vi "create_method.vi"(0 "template_path":path=path "C:/Users/hugoc/TDF Dropbox/2_Technologies de France/1 - Services et Etudes/_Missions/HC/6 - PLAIYLAB/code/Model/_Template/common/specific_data/fit.vit", 5 "ModuleModelFunction":string[](array[string])=["tree", "DecisionTreeClassifier", "fit"], 7 "Control Path":path=path "C:/Users/hugoc/TDF Dropbox/2_Technologies de France/1 - Services et Etudes/_Missions/HC/6 - PLAIYLAB/code/Model/Supervised/Tree/Tree.lvclass", 9 "Path to Saved File":path, 11 "error in (no error)":errorcluster, 12 "Parameters?":bool) -> (15 "error out":errorcluster)   [LabVIEW 2020]
doc: "Create a method based on a template with the correct documentation."
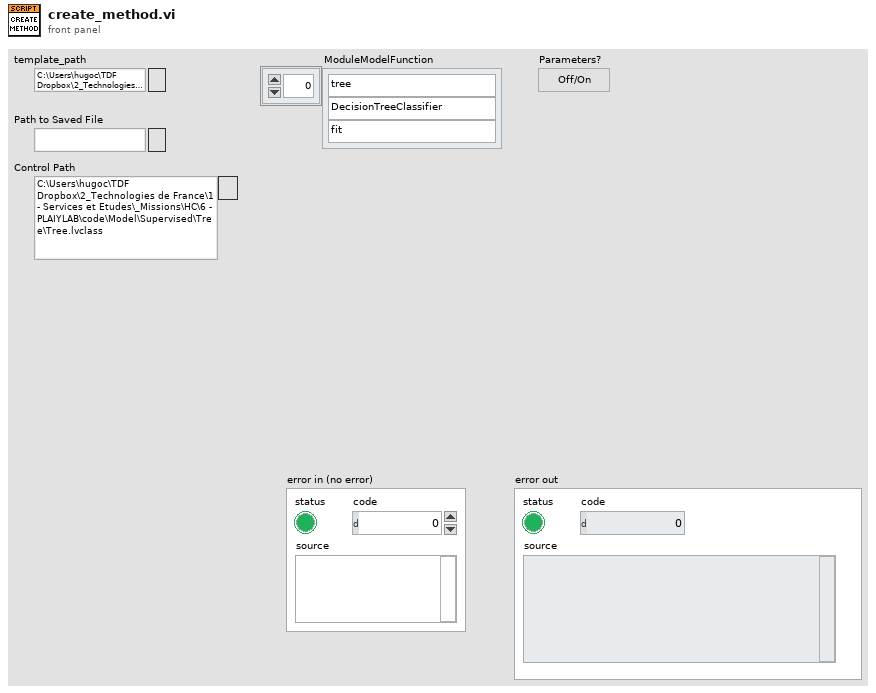
[diagram p1: front panel]
types:
  T1 = enum32{"invalid VI type", "Standard VI", "Control VI", "Global VI", "Polymorphic VI", "Configuration VI", "SubSystem", "Facade VI", "Method VI", "Statechart Diagram VI"}
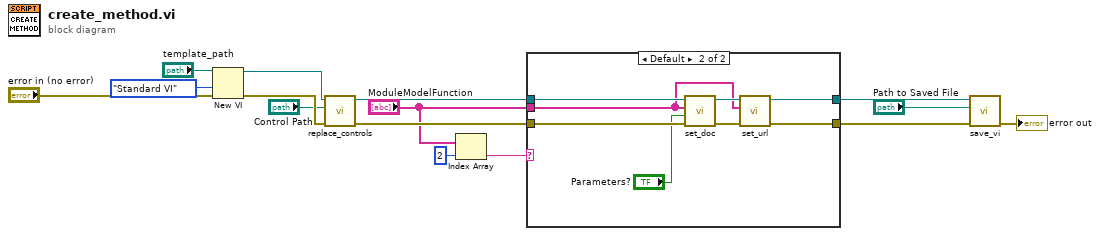
[diagram p0: block diagram]
diagram:
  n1 = New VI(8:"error in (no error)", 9:T1."Standard VI" ("vi type (standard vi)"), 10:"template_path") -> (0:w14:errorcluster, 3:w12:refnum<vi>)  [unwired: 4 in]
  n2 = call "replace_controls.vi"("error in (no error)"=w14, "Path to new control"="Control Path", "VI in"=w12) -> ("error out"=w10:errorcluster, "VI out"=w9:refnum<vi>)  [unwired: 7 in]
  n3 = Index Array(array="ModuleModelFunction", index=2) -> (element=w1:string)
  n4 = case shown="Default" w1 {
    tunnel: w10 -> [w16 w25]
    tunnel: w9 -> [w17 w23]
    tunnel: [w17 w21] -> w8
    tunnel: [w16 w20] -> w7
    tunnel: "ModuleModelFunction" -> [_ w18]
    frame "get_attributes", "get_params", "set_params" {
    }
    frame Default {
      n5 = call "set_doc.vi"("error in"=w25, "Parameters?"="Parameters?", "Array"=w18, "vi refnum"=w23) -> ("error out"=w19:errorcluster, "reference out"=w22:refnum<vi>)  [unwired: 6 in]
      n6 = call "set_url.vi"("error in (no error)"=w19, "Array in"=w18, "VI in"=w22) -> ("error out"=w20:errorcluster, "VI out"=w21:refnum<vi>)  [unwired: 7 in]
    }
  }
  n7 = call "save_vi.vi"("error in (no error)"=w7, "Path to Saved File"="Path to Saved File", "VI in"=w8) -> ("error out"=→"error out":errorcluster)  [unwired: 8 in]
